vi "AlliGator Get Message & Parameters from JSON Output.vi"(8 "error in (no error)":errorcluster, 9 "Function Display Name":string, 11 "<JSON>":string) -> (0 "error out":errorcluster, 3 "Notebook Message":string)   [LabVIEW 2021, in "AlliGator Python Plugins.lvlib"]
doc: "Interprets JSON string output and formats it to be sent to the Notebook."
uses:
  AlliGator Python Plugins.lvlib
  e740c2e0-9a90-4bfa-a972-264106710fde.vi
  be866606-4d0a-45f1-ac73-4d3dc2d14972.vi
  52e5e8cd-1212-47aa-b53a-cd2c4881839b.vi
  <vilib>/JDP Science/JSONtext/JSON text to Variant.vi
  <vilib>/JDP Science/JSONtext/LVClass Serializer/JSONtext LVClass Serializer.lvclass
  <vilib>/JDP Science/JSONtext/JSONtext.lvlib
  Strings/Strings.lvlib
  AlliGator Settings.lvlib
panel:
  # "see the AlliGator License on the block diagram (Ctrl+E or Window:Show Block Diagram)"
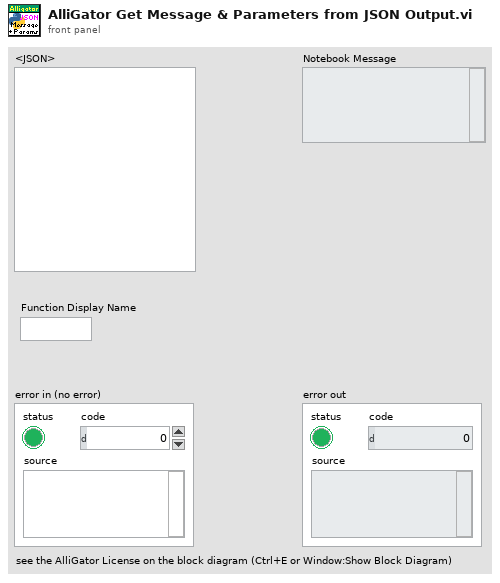
[diagram p1: front panel]
types:
  T1 = typedef "AlliGator Settings.lvlib/AlliGator Settings List.ctl" = enum16{"GUI:Visible Settings Tab", "GUI:Last Run Version", "Source Image:Use Image Histogram for Contrast", "Source Image:Low Count Pixels Rejection Options", "Source Image:High Count Pixels Rejection Options", "Source Image:Use Image Brightness", "Source Image:Blend Overlay with Image Background", "Source Image:Use Fixed ROI Diameter", "Source Image:ROI Diameter", "Source Image:ROI Center Color", "Source Image:Peak Threshold", "Source Image:Intensity Threshold", "Source Image:Image Binning Options", "Source Image:Image Smoothing Options", "Source Image:Image Histogram Active", "Source Image:Invert Binary Mask", "Source Image:Hot Pixel Removal", "Source Image:Overlay Analyzed ROI Center", "Source Image:Auto-Adjust Contrast", "Source Image:Histogram Lower Percentile", "Source Image:Histogram Upper Percentile", "Source Image:Save Source Image", "Source Image:Scale Bar Options", "Source Image:Image Resolution (Pixel Size)", "Source Image:Flatfield Correction", "Source Image:Show Dead Left Columns Correction", "Source Image:Dead Left Columns Correction", "Source Image:Image Pre-Processing Operations Order", "Source Image:Overlay ROI Median", "Source Image:Median Overlay Color", "Data Information:Gate Width", "Data Information:Nanotime Gate Separation", "Data Information:Macrotime Gate Separation", "Data Information:Gate Step", "Data Information:# Gates", "Data Information:Gate Image Exposure", "Data Information:Gate Image Integration", "Data Information:Gates to Skip", "Data Information:Gates to Keep", "Data Information:Define Gates to", "Data Information:Channel Name", "Data Information:Available Channel Names", "Data Information:Channel Arithmetic", "Data Information:Background File Subtraction", "Data Information:Background File", "Data Information:Background Scaling Factor", "Data Information:Background Pile-up Correction", "Data Information:Background Pixel Well Capacity", "Data Information:Laser Period", "Data Information:SYNC Period", "Data Information:Pile-up Correction", "Data Information:Pixel Well Capacity", "Data Information:Dataset Scaling Factor", "Fluorescence Decay_Decay Pre-Processing:Reverse Gates", "Fluorescence Decay_Decay Pre-Processing:Verbose Decay Pre-Processing", "Fluorescence Decay_Decay Pre-Processing:Use Decay Pre-Processing", "Fluorescence Decay_Decay Pre-Processing:Background Subtraction", "Fluorescence Decay_Decay Pre-Processing:Background Definition Range", "Fluorescence Decay_Decay Pre-Processing:Baseline Subtraction Method", "Fluorescence Decay_Decay Pre-Processing:Decay Pre-Processing Operations Order", "Fluorescence Decay_Decay Pre-Processing:Smoothing Parameter", "Fluorescence Decay_Decay Pre-Processing:Shift Decay", "Fluorescence Decay_Decay Pre-Processing:Decay Shift Parameters", "Fluorescence Decay_Decay Pre-Processing:Fold Decay", "Fluorescence Decay_Decay Pre-Processing:# Folds", "Fluorescence Decay_Decay Pre-Processing:1-Normalize Decay", "Fluorescence Decay_Decay Pre-Processing:[0-1]-Normalize Decay", "Fluorescence Decay_Decay Pre-Processing:Smoothen Decay", "Fluorescence Decay_Decay Pre-Processing:Extrapolate Decay", "Fluorescence Decay_Decay Pre-Processing:Use Periodicity", "Fluorescence Decay_Decay Pre-Processing:Use Cursors", "Fluorescence Decay_Decay Pre-Processing:Tail Fraction", "Fluorescence Decay_Decay Pre-Processing:Head Fraction", "Fluorescence Decay_Decay Pre-Processing:Additional Points", "Fluorescence Decay_Decay Pre-Processing:Straighten Decay", "Fluorescence Decay_Decay Pre-Processing:Constant Background", "Fluorescence Decay_Decay Pre-Processing:Pixel-Normalize Decay", "Fluorescence Decay_Advanced Analysis:Extract IRF instead of Decay", "Fluorescence Decay_Advanced Analysis:IRF Extraction Options", "Fluorescence Decay_Advanced Analysis:IRF Optimization Options", "Fluorescence Decay_Advanced Analysis:Square Pulse Options", "Fluorescence Decay_Advanced Analysis:IRF Order", "Fluorescence Decay_Advanced Analysis:IRF Time Constants", "Fluorescence Decay_Advanced Analysis:Wavelet Analysis Options", "Fluorescence Decay_Advanced Analysis:Average Lifetime Options", "Fluorescence Decay_Fit Options:Fit Options", "Fluorescence Decay_Fit Options:Use Legacy Fitting Approach", "Fluorescence Decay_Fit Options:Use Data Information Laser Period", "Fluorescence Decay_Fit Parameters:Displayed Fit Parameters", "Fluorescence Decay_Fit Parameters:Fit Parameter Constraints", "Fluorescence Decay_Fit Parameters:Export Tabulated Results", "Fluorescence Decay_Fit Parameters:MLE Baseline Offset Type", "Fluorescence Decay_Fit Parameters:MLE Baseline Offset", "Fluorescence Decay_Fit Parameters:Guess Parameter Names", "Fluorescence Decay_Fit Parameters:Guess Parameter Values", "Fluorescence Decay_Fit Parameters:Guess Parameters Options", "Fluorescence Decay_Styles:Show Last Decay Only", "Fluorescence Decay_Styles:Decay Graph Color Array", "Fluorescence Decay:Decay Graph Active", "Fluorescence Decay Statistics:Min Peak Value", "Fluorescence Decay Statistics:Reject Low Decay Peak Pixels", "Fluorescence Decay Statistics:Reject High Decay Peak Pixels", "Fluorescence Decay Statistics:Max Peak Value", "Time Traces:Use File Timestamp", "Time Traces:Time Step", "Time Traces:Use Intensity Correction File", "Time Traces:Intensity Correction File", "Phasor Plot:Phasor Plot Smoothing Options", "Phasor Plot:Phasor Plot Size", "Phasor Plot:Phasor Plot Graphics Options", "Phasor Plot:Cumulative Phasor Plot", "Phasor Plot:Use Phasor Brightness", "Phasor Plot:Blend Overlay with Phasor Background", "Phasor Plot:Save Phasor Plot", "Phasor Plot:Show References", "Phasor Plot:Phasor Ratio Decay Range", "Phasor Plot:Exponential Fading", "Phasor Plot:Phasor Ratio Reference Colors", "Phasor Plot:Reference Radius", "Phasor Plot:Show Color Map Vertices", "Phasor Plot:Phasor Plot Active", "Phasor Plot:Phasor Ratio Color Map Type", "Phasor Plot:Phasor Ratio Color Map", "Phasor Plot:Phasor Ratio Display Range", "Phasor Plot:Selected Image ROI(s)", "Phasor Plot:All Image ROIs", "Phasor Plot:Selected Phasor Plot ROI(s)", "Phasor Plot:All Phasor Plot ROIs", "Phasor Plot:Phasor Ratio Color-Coded Quantity", "Phasor Plot:Store Phasor Harmonics", "Phasor Plot:Draw Reference Segment", "Phasor Plot:User-Defined Quantity", "Phasor Graph:Phasor Frequency", "Phasor Graph:Phasor Ratio Type", "Phasor Graph:Pixel-level Phasor Computation", "Phasor Graph:Save Phasor Graph", "Phasor Graph:Phasor Graph Active", "Phasor Graph:Phasor SDV Options", "Phasor Calibration:Use Backup Calibration if needed", "Phasor Graph:Define Shortest Lifetime as", "Phasor Calibration:Backup Calibration Type", "Phasor Calibration:Calibration Type", "Phasor Calibration:Calibration Lifetime", "Phasor Calibration:Calibration Map Algorithm", "Single-Exponential Phasor Locus (SEPL):Gate Parameters", "Single-Exponential Phasor Locus (SEPL):User-defined Gate", "Single-Exponential Phasor Locus (SEPL):User-defined IRF", "Single-Exponential Phasor Locus (SEPL):Phasor Parameters", "Single-Exponential Phasor Locus (SEPL):Decay & IRF Parameters", "Single-Exponential Phasor Locus (SEPL):Display Parameters", "Lifetime Analysis:Decay Analysis Parameters", "Lifetime Analysis:Lifetime Map Active", "Plugins:Python Settings", "Miscellaneous:Verbose Mode", "Miscellaneous:Beep after Script", "Miscellaneous:Saved Image File Format", "Miscellaneous:Exported Gate Image Settings", "Miscellaneous:Include Loading in Timing", "Miscellaneous:Verbose Settings Mode", "Miscellaneous:Histogram Options", "Miscellaneous:Beep on Error", "Miscellaneous:# Logical Processors Used", "Miscellaneous:ROI Description Max Characters", "Miscellaneous:Verbose Error Mode", "Miscellaneous:Transparent Mask Color"}
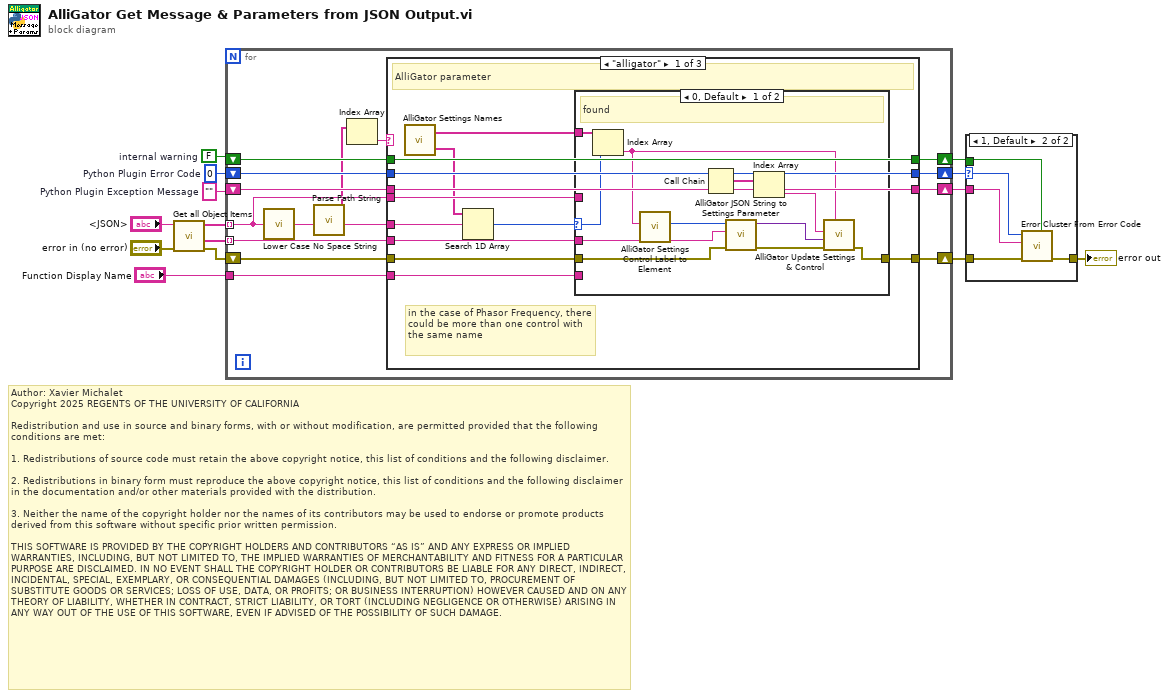
[diagram p0: block diagram]
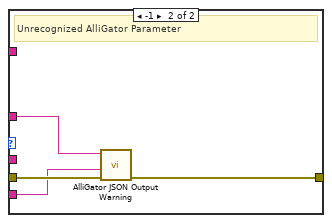
[diagram p2: hidden frame]
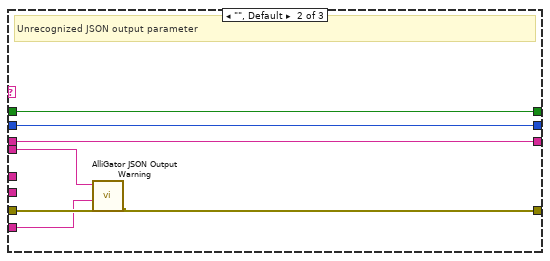
[diagram p3: hidden frame]
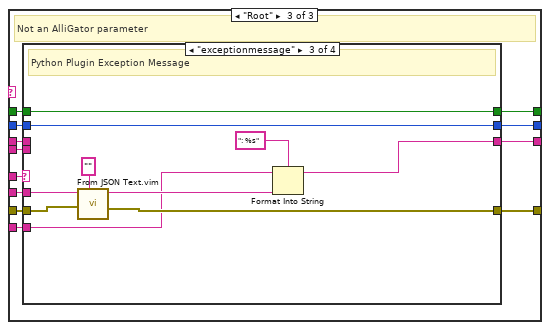
[diagram p4: hidden frame]
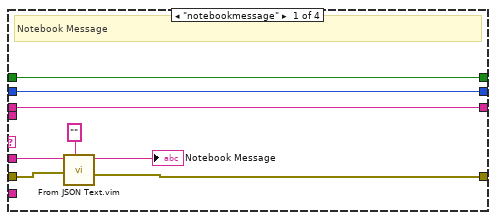
[diagram p5: hidden frame]
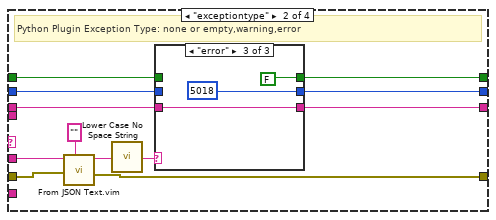
[diagram p6: hidden frame]
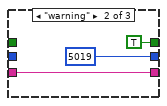
[diagram p8: hidden frame]
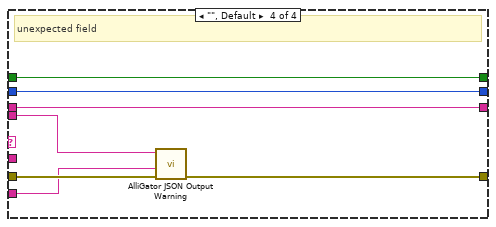
[diagram p9: hidden frame]
diagram:
  w1 = ""  # Python Plugin Exception Message
  w2 = FALSE  # internal warning
  w3 = 0  # Python Plugin Error Code
  # "Author: Xavier Michalet\nCopyright 2025 REGENTS OF THE UNIVERSITY OF CALIFORNIA\n\nRedistribution and use in source and binary forms, with or without modification, are permitted provided that the following conditions are met:\n\n1. Redistributions of source code must retain the above copyright notice, this list of conditions and the following disclaimer.\n\n2. Redistributions in binary form must reproduce the above copyright notice, this list of conditions and the following disclaimer in the documentation and/or other materials provided with the distribution.\n\n3. Neither the name of the copyright holder nor the names of its contributors may be used to endorse or promote products derived from this software without specific prior written permission.\n\nTHIS SOFTWARE IS PROVIDED BY THE COPYRIGHT HOLDERS AND CONTRIBUTORS “AS IS” AND ANY EXPRESS OR IMPLIED WARRANTIES, INCLUDING, BUT NOT LIMITED TO, THE IMPLIED WARRANTIES OF MERCHANTABILITY AND FITNESS FOR A PARTICULAR PURPOSE ARE DISCLAIMED. IN NO EVENT SHALL THE COPYRIGHT HOLDER OR CONTRIBUTORS BE LIABLE FOR ANY DIRECT, INDIRECT, INCIDENTAL, SPECIAL, EXEMPLARY, OR CONSEQUENTIAL DAMAGES (INCLUDING, BUT NOT LIMITED TO, PROCUREMENT OF SUBSTITUTE GOODS OR SERVICES; LOSS OF USE, DATA, OR PROFITS; OR BUSINESS INTERRUPTION) HOWEVER CAUSED AND ON ANY THEORY OF LIABILITY, WHETHER IN CONTRACT, STRICT LIABILITY, OR TORT (INCLUDING NEGLIGENCE OR OTHERWISE) ARISING IN ANY WAY OUT OF THE USE OF THIS SOFTWARE, EVEN IF ADVISED OF THE POSSIBILITY OF SUCH DAMAGE."
  n1 = call <vilib>:"Get all Object Items.vi"("error in (no error)"="error in (no error)", "JSON"="<JSON>") -> ("error out"=w12:errorcluster, "<JSON>"=w11:string[], "Item Names"=w10:string[])  [unwired: 6 in, 1 out]
  n2 = for {
    tunnel: w10 -> [w26] mode=indexing
    tunnel: w11 -> [w29] mode=indexing
    shift-right: [w27] -> w13
    shift-left: w12 -> [w28]
    tunnel: "Function Display Name" -> [w25]
    shift-right: [w24] -> w6
    shift-left: w2 -> [w20]
    shift-right: [w23] -> w5
    shift-left: w3 -> [w19]
    shift-right: [w22] -> w4
    shift-left: w1 -> [w21]
    n3 = call "Lower Case No Space String.vi"("String"=w26) -> ("Lower Case No Space String"=w18:string)
    n4 = call "Parse Path String.vi"("Path in"=w18) -> ("Folder Hierarchy"=w16:string[], "File/Folder"=w17:string)  [unwired: 4 in]
    n5 = Index Array(array=w16) -> (element=w15:string)  [unwired: 1 in]
    n6 = case shown="\"alligator\"" w15 {
      tunnel: w29 -> [w34 _ w75]
      tunnel: w28 -> [w38 w63 w74]
      tunnel: [w35 w60 w73] -> w27
      tunnel: w26 -> [w37 w61 w72]
      tunnel: w25 -> [w36 w62 w71]
      tunnel: [w41 w59 w70] -> w24
      tunnel: [w40 w58 w69] -> w23
      tunnel: [w39 w57 w68] -> w22
      tunnel: w21 -> [w39 w57 w67]
      tunnel: w20 -> [w41 w59 w66]
      tunnel: w19 -> [w40 w58 w65]
      tunnel: w17 -> [w31 _ w64]
      frame "alligator" {
        # "in the case of Phasor Frequency, there could be more than one control with the same name"
        # "AlliGator parameter"
        n7 = call "AlliGator Settings Names.vi"() -> ("Settings Name Array (lower case no space)"=w32:string[], "Settings Name Array"=w33:string[])  [unwired: 2 in]
        n8 = Search 1D Array(1D array=w32, element=w31) -> (index of element=w30:i32)  [unwired: 1 in]
        n9 = case shown="0, Default" w30 {
          selector: w30 -> [w52 _]
          tunnel: w38 -> [w44 w56]
          tunnel: w37 -> [_ w55]
          tunnel: w36 -> [_ w54]
          tunnel: [w50 w53] -> w35
          tunnel: w33 -> [w51 _]
          tunnel: w34 -> [w45 _]
          frame 0, Default {
            # "found"
            n10 = Index Array(array=w51, index=w52) -> (element=w47:string)
            n11 = call "AlliGator Settings Control Label to Element.vi"("Control Label"=w47) -> ("AlliGator Settings List Element"=w46:T1)  [unwired: 7 in, 1 out]
            n12 = Call Chain() -> (call chain=w49:string[])
            n13 = call "AlliGator JSON String to Settings Parameter.vi"("error in (no error)"=w44, "<JSON>"=w45, "AlliGator Settings List Element"=w46) -> ("error out"=w43:errorcluster, "Variant"=w42:variant)  [unwired: 7 in]
            n14 = Index Array(array=w49) -> (element=w48:string)  [unwired: 1 in]
            n15 = call "AlliGator Update Settings & Control.vi"("Control Label"=w47, "Error In"=w43, "Value"=w42, "Sender"=w48) -> ("Error Out"=w50:errorcluster)  [unwired: 7 in]
          }
          frame -1 {
            # "Unrecognized AlliGator Parameter"
            n16 = call "AlliGator JSON Output Warning.vi"("error in (no error)"=w56, "Function Name"=w54, "JSON Element Name"=w55) -> ("error out"=w53:errorcluster)  [unwired: 8 in]
          }
        }
      }
      frame "", Default {
        # "Unrecognized JSON output parameter"
        n17 = call "AlliGator JSON Output Warning.vi"("error in (no error)"=w63, "Function Name"=w62, "JSON Element Name"=w61) -> ("error out"=w60:errorcluster)  [unwired: 8 in]
      }
      frame "Root" {
        # "Not an AlliGator parameter"
        n18 = case shown="\"exceptionmessage\"" w64 {
          tunnel: w75 -> [w83 w95 w114 _]
          tunnel: w74 -> [w81 w94 w113 w121]
          tunnel: [w80 w86 w109 w120] -> w73
          tunnel: w72 -> [_ _ _ w119]
          tunnel: w71 -> [_ _ w106 w118]
          tunnel: [w78 w93 w111 w117] -> w70
          tunnel: [w77 w92 w110 w116] -> w69
          tunnel: [w76 w89 w108 w115] -> w68
          tunnel: w67 -> [w76 w90 _ w115]
          tunnel: w66 -> [w78 w88 w111 w117]
          tunnel: w65 -> [w77 w87 w110 w116]
          frame "notebookmessage" {
            # "Notebook Message"
            n19 = call "From JSON Text.vim"("Data Type and Default Value"="" ("Message"), "error in (no error)"=w81, "JSON"=w83) -> ("error out"=w80:errorcluster, "Data out"=→"Notebook Message":string)  [unwired: 7 in]
          }
          frame "exceptiontype" {
            # "Python Plugin Exception Type: none or empty,warning,error"
            n20 = call "From JSON Text.vim"("Data Type and Default Value"="" ("Message"), "error in (no error)"=w94, "JSON"=w95) -> ("error out"=w86:errorcluster, "Data out"=w85:string)  [unwired: 7 in]
            n21 = call "Lower Case No Space String.vi"("String"=w85) -> ("Lower Case No Space String"=w84:string)
            n22 = case shown="\"error\"" w84 {
              tunnel: [w98 TRUE ("is warning? (False)") FALSE ("is warning? (False)")] -> w93
              tunnel: [w97 5019 ("error code (0)") 5018 ("error code (0)")] -> w92
              tunnel: w90 -> [w96 w101 w102]
              tunnel: [w96 w101 w102] -> w89
              tunnel: w88 -> [w98 _ _]
              tunnel: w87 -> [w97 _ _]
              frame "", Default {
              }
              frame "warning" {
              }
              frame "error" {
              }
            }
          }
          frame "exceptionmessage" {
            # "Python Plugin Exception Message"
            n23 = call "From JSON Text.vim"("Data Type and Default Value"="" ("Message"), "error in (no error)"=w113, "JSON"=w114) -> ("error out"=w109:errorcluster, "Data out"=w107:string)  [unwired: 7 in]
            n24 = Format Into String(format string=": %s", initial string=w106, w107) -> (resulting string=w108:string)  [unwired: 1 in, 1 out]
          }
          frame "", Default {
            # "unexpected field"
            n25 = call "AlliGator JSON Output Warning.vi"("error in (no error)"=w121, "Function Name"=w118, "JSON Element Name"=w119) -> ("error out"=w120:errorcluster)  [unwired: 8 in]
          }
        }
      }
    }
  }
  n26 = case shown="1, Default" w5 {
    selector: w5 -> [_ w124]
    tunnel: w13 -> [w122 w127]
    tunnel: [w122 w126] -> w7
    tunnel: w6 -> [_ w125]
    tunnel: w4 -> [_ w123]
    frame 0 {
    }
    frame 1, Default {
      n27 = call <vilib>:"Error Cluster From Error Code.vi"("is warning? (False)"=w125, "error in (no error)"=w127, "error message (\"\")"=w123, "error code (0)"=w124) -> ("error out"=w126:errorcluster)  [unwired: 5 in]
    }
  }
  "error out" <- w7
